vi "SetTriggerPointMeasurement.vi"(8 "error in":errorcluster) -> (0 "error out":errorcluster)   [LabVIEW 2011]
uses:
  <vilib>/DAQmx/write.llb/DAQmx Write (Digital Bool 1Line 1Point).vi
  <vilib>/DAQmx/create/channels.llb/DAQmx Create Channel (DO-Digital Output).vi
  <vilib>/DAQmx/miscellaneous.llb/DAQmx Fill In Error Info.vi
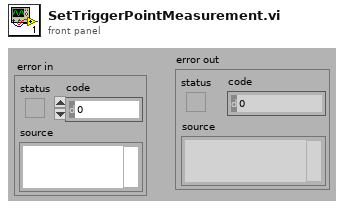
[diagram p1: front panel]
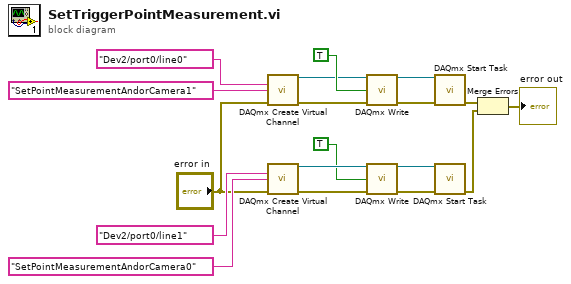
[diagram p0: block diagram]
diagram:
  n1 = call-poly <vilib>:"DAQmx Create Virtual Channel.vi"("lines"=tag "Dev2/port0/line0" ("lines 2"), "name to assign"="SetPointMeasurementAndorCamera1", "error in"="error in") -> ("task out"=w10:refnum<k21>, "error out"=w9:errorcluster)  [unwired: 11 in]
  n2 = call-poly <vilib>:"DAQmx Create Virtual Channel.vi"("lines"=tag "Dev2/port0/line1", "name to assign"="SetPointMeasurementAndorCamera0", "error in"="error in") -> ("task out"=w18:refnum<k21>, "error out"=w17:errorcluster)  [unwired: 11 in]
  n3 = call-poly <vilib>:"DAQmx Write.vi"("task/channels in"=w10, "data"=TRUE, "error in"=w9) -> ("task out"=w1:refnum<k21>, "error out"=w5:errorcluster)  [unwired: 10 in, 1 out]
  n4 = call-poly <vilib>:"DAQmx Write.vi"("task/channels in"=w18, "data"=TRUE, "error in"=w17) -> ("task out"=w13:refnum<k21>, "error out"=w12:errorcluster)  [unwired: 10 in, 1 out]
  n5 = call <vilib>:"DAQmx Start Task.vi"("task/channels in"=w1, "error in"=w5) -> ("error out"=w4:errorcluster)  [unwired: 12 in, 1 out]
  n6 = call <vilib>:"DAQmx Start Task.vi"("task/channels in"=w13, "error in"=w12) -> ("error out"=w3:errorcluster)  [unwired: 12 in, 1 out]
  n7 = Merge Errors(w4, w3) -> (→"error out":errorcluster)
